vi "Update Flow Graph Point and Flow Alarm.vi"(1 "Current Step ID":i32, 3 "Actual Flow vs Current":cluster{dbl, dbl}, 4 "Low Flow Limit vs Current":cluster{"Min":dbl, dbl}, 5 "High Flow Limit vs Current":cluster{"Min":dbl, dbl}) -> ()   [LabVIEW 2018]
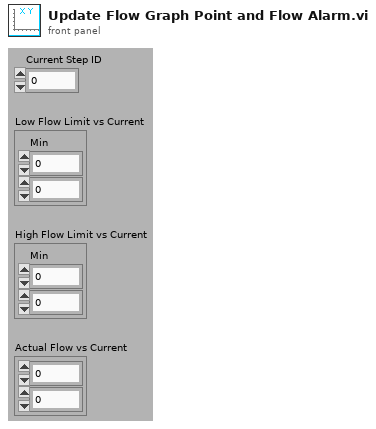
[diagram p1: front panel]
types:
  T1 = enum16{"get data", "set data", "Add Data Pair", "initialize"}
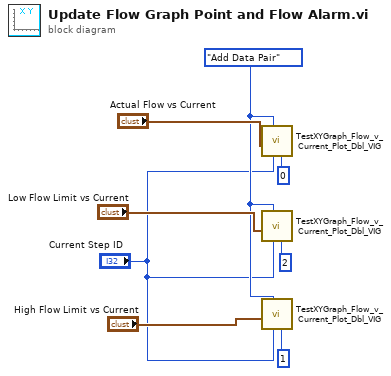
[diagram p0: block diagram]
diagram:
  w2 = T1."Add Data Pair" ("Operation")
  n1 = call "TestXYGraph_Flow_v_Current_Plot_Dbl_VIG.vi"("Plot Index/Size"=0, "Point index/size"="Current Step ID", "Operation"=w2, "XY Point"="Actual Flow vs Current") -> ()  [unwired: 5 in, 3 out]
  n2 = call "TestXYGraph_Flow_v_Current_Plot_Dbl_VIG.vi"("Plot Index/Size"=2, "Point index/size"="Current Step ID", "Operation"=w2, "XY Point"="Low Flow Limit vs Current") -> ()  [unwired: 5 in, 3 out]
  n3 = call "TestXYGraph_Flow_v_Current_Plot_Dbl_VIG.vi"("Plot Index/Size"=1, "Point index/size"="Current Step ID", "Operation"=w2, "XY Point"="High Flow Limit vs Current") -> ()  [unwired: 5 in, 3 out]
